vi "Configure Power.vi"(8 "error in (no error)":errorcluster, 10 "Power [dBm]":dbl, 11 "VNA-CMT S2 S4 in":refnum<class "VNA-CMT S2 S4.lvclass">) -> (0 "error out":errorcluster, 3 "VNA-CMT S2 S4 out":refnum<class "VNA-CMT S2 S4.lvclass">)   [LabVIEW 2020, in "VNA-CMT S2 S4.lvclass"]
doc: "Configure the output power.\nThe power will be corrected to the nearest supported."
uses:
  VNA-CMT S2 S4.lvclass
  C:/Sandbox/Git_Sandbox/WiSpry Test Framework source code (LV20)/WiSpry Test Framework/Instruments/Instrument.lvclass
  Instrument.lvclass/Instrument.ctl
  Instrument.lvclass
  <instrlib>/CMT S2 and S4 VNA/CMT S2 and S4 VNA.lvlib
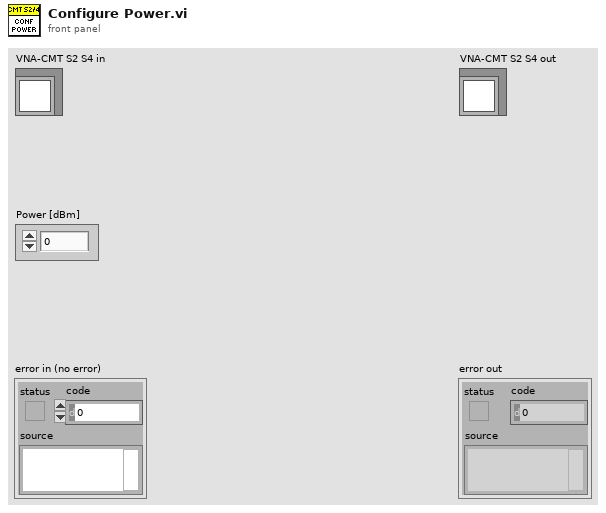
[diagram p1: front panel]
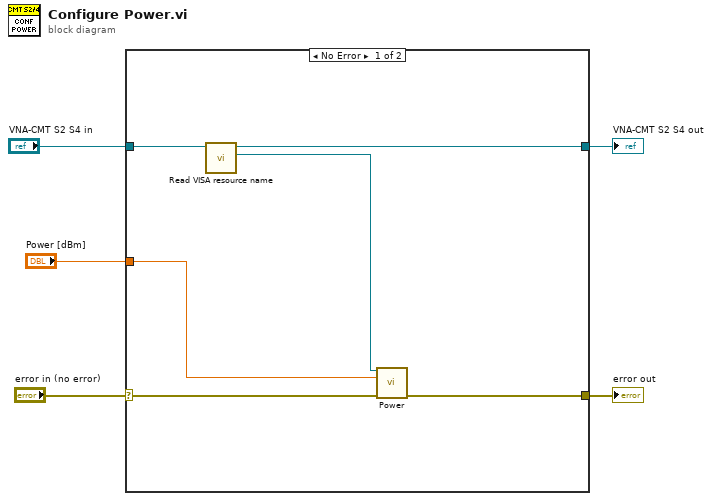
[diagram p0: block diagram]
diagram:
  n1 = case shown="No Error" "error in (no error)" {
    selector: "error in (no error)" -> [w7 w12]
    tunnel: "VNA-CMT S2 S4 in" -> [w11 w13]
    tunnel: [w10 w13] -> w3
    tunnel: [w6 w12] -> w4
    tunnel: "Power [dBm]" -> [w8 _]
    frame No Error {
      n2 = call "Read VISA resource name.vi"("Instrument in"=w11) -> ("VISA resource name"=w9:refnum<visa-resource-name>, "Instrument out"=w10:refnum<class "VNA-CMT S2 S4.lvclass">)  [unwired: 9 in]
      n3 = call <instrlib>:"Power.vi"("VISA resource name"=w9, "Power Level (0.0)"=w8, "error in (no error)"=w7) -> ("error out"=w6:errorcluster)  [unwired: 11 in, 1 out]
    }
    frame Error {
    }
  }
  "error out" <- w4
  "VNA-CMT S2 S4 out" <- w3
